vi "request.From JSON Tree.vi"(8 "error in (no error)":errorcluster, 10 "JSON Value in":variant, 11 "Request in":refnum<class "Request.lvclass">) -> (0 "error out":errorcluster, 3 "Request out":refnum<class "Request.lvclass">)   [LabVIEW 2017, in "Request.lvclass"]
uses:
  Request.lvclass
  params/params.lvclass
  id/id.lvclass
  Request.lvclass/Request.ctl
  <vilib>/National Instruments/Variant Data Manipulation/Variant Data Manipulation.lvlib
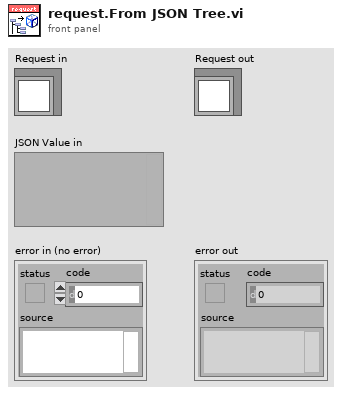
[diagram p1: front panel]
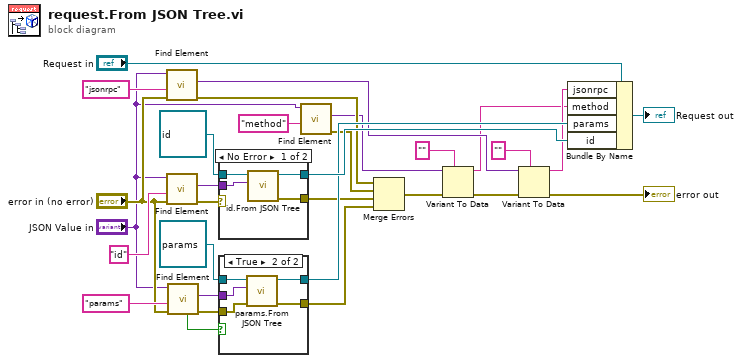
[diagram p0: block diagram]
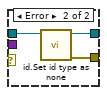
[diagram p3: hidden frame]
diagram:
  n1 = call <vilib>:"Find Element.vi"("error in (no error)"="error in (no error)", "Name"="jsonrpc" ("Parameter Name"), "Variant (Cluster) in"="JSON Value in") -> ("error out"=w18:errorcluster, "element"=w11:variant)  [unwired: 4 in, 3 out]
  n2 = call <vilib>:"Find Element.vi"("error in (no error)"="error in (no error)", "Name"="id" ("Parameter Name"), "Variant (Cluster) in"="JSON Value in") -> ("error out"=w13:errorcluster, "element"=w14:variant)  [unwired: 4 in, 3 out]
  n3 = call <vilib>:"Find Element.vi"("error in (no error)"="error in (no error)", "Name"="params" ("Parameter Name"), "Variant (Cluster) in"="JSON Value in") -> ("error out"=w1:errorcluster, "element"=w15:variant, "found?"=w2:bool)  [unwired: 4 in, 2 out]
  n4 = case shown="No Error" w13 {
    tunnel: refnum<class "id.lvclass"> refnum ("id.lvclass") -> [w34 w37]
    tunnel: w14 -> [w33 _]
    tunnel: [w32 w36] -> w27
    tunnel: [w31 w35] -> w24
    frame No Error {
      n5 = call "id.From JSON Tree.vi"("JSON Value in"=w33, "id in"=w34) -> ("error out"=w31:errorcluster, "id out"=w32:refnum<class "id.lvclass">)  [unwired: 8 in]
    }
    frame Error {
      n6 = call "id.Set id type as none.vi"("id in"=w37) -> ("error out"=w35:errorcluster, "id out"=w36:refnum<class "id.lvclass">)  [unwired: 9 in]
    }
  }
  n7 = case shown="True" w2 {
    tunnel: refnum<class "params.lvclass"> refnum ("params.lvclass") -> [w39 w44]
    tunnel: w15 -> [_ w43]
    tunnel: [w39 w42] -> w25
    tunnel: [w38 w41] -> w19
    tunnel: w1 -> [w38 w40]
    frame False {
    }
    frame True {
      n8 = call "params.From JSON Tree.vi"("error in (no error)"=w40, "JSON Value in"=w43, "params in"=w44) -> ("error out"=w41:errorcluster, "params in"=w42:refnum<class "params.lvclass">)  [unwired: 7 in]
    }
  }
  n9 = call <vilib>:"Find Element.vi"("Name"="method" ("Parameter Name"), "Variant (Cluster) in"="JSON Value in") -> ("error out"=w17:errorcluster, "element"=w8:variant)  [unwired: 5 in, 3 out]
  n10 = Merge Errors(w18, w17, w24, w19) -> (w5:errorcluster)
  n11 = Variant To Data(error in=w5, type="" ("Parameter Name"), Variant=w8) -> (data=w6:string, error out=w4:errorcluster)
  n12 = Variant To Data(error in=w4, type="" ("Parameter Name"), Variant=w11) -> (data=w9:string, error out=→"error out":errorcluster)
  n13 = Bundle By Name(cluster="Request in", "jsonrpc"=w9, "method"=w6, "params"=w25, "id"=w27) -> (→"Request out":refnum<class "Request.lvclass">)
